vi "AmplitudeLinear_Log.vi"() -> ()   [LabVIEW 2020]
panel:
  out "Waveform Graph":dbl[](graph)
  in  "Enum":enum16{"Linear", "Logarithmic Base10"}(ring)
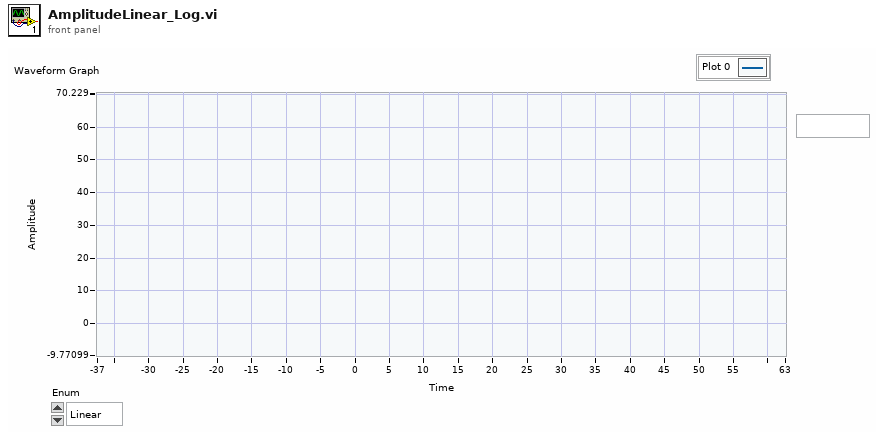
[diagram p1: front panel]
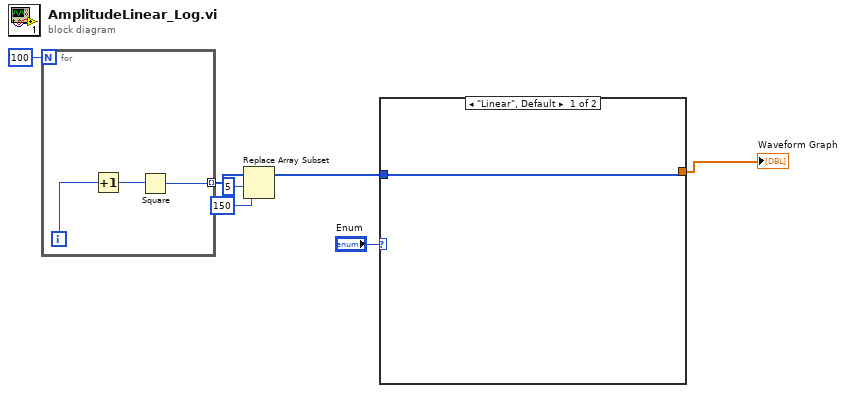
[diagram p0: block diagram]
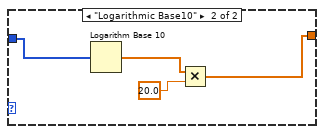
[diagram p2: hidden frame]
diagram:
  n1 = for {
    N: 100 -> [_]
    tunnel: [w8] -> w5 mode=indexing
    i -> [w9]
    n2 = Increment(x=w9) -> (x+1=w10:i32)
    n3 = Square(x=w10) -> (x^2=w8:i32)
  }
  n4 = Replace Array Subset(array=w5, new element=150 ("new element/subarray"), index=5) -> (w2:i32[])
  n5 = case shown="\"Linear\", Default" "Enum" {
    tunnel: w2 -> [w11 w15]
    tunnel: [w11 w12] -> w1
    frame "Linear", Default {
    }
    frame "Logarithmic Base10" {
      n6 = Logarithm Base 10(1:w15) -> (0:w14:dbl[])
      n7 = Multiply(x=w14, y=20.0) -> (x*y=w12:dbl[])
    }
  }
  "Waveform Graph" <- w1
